vi "DVS_LabVIEWController_april2015 - Copy.vi"() -> ()   [LabVIEW 2013]
doc: "This example demonstrates temperature control and monitoring.\n\nNote:\nBefore start this VI is it necessary:\n\n- preconfigure some specific parameters that are not supported by this driver (e.g. PV-I/O Type, Linearization type, Alarm Input Values... ) by Quick Codes, or by Eurotherm iTools or by instrument front panel controls\n- enter correct VISA Resource Descriptor, Device Address and Baud Rate into front-panel controls"
uses:
  <vilib>/Utility/file.llb/Write To Spreadsheet File (string).vi
  <vilib>/Instr/_visa.llb/VISA Configure Serial Port (Instr).vi
  <instrlib>/Keithley 6430/Public/Data/Read (Single Point).vi
  <instrlib>/Keithley 24XX/Public/Data/Read (Single Point).vi
  <instrlib>/Keithley 24XX/Keithley 24XX.lvlib
  <instrlib>/Keithley 6430/Keithley 6430.lvlib
panel:
  out "(Ohm)":dbl format="%^_7e"
  out "Waveform Chart 9":cluster{"Measurement":dbl}(graph)
  in  "Keithley 6430":bool
  in  "Keithley 2422":bool
  in  "Keithley 2423":bool
  in  "Keithley 2421":bool
  in  "stop":bool
  in  "Keithley 2420":bool
  in  "J-KEM":bool
  out "Start Time":string
  out "Elapsed (min)":dbl caption="Elapsed Time (s)"
  out "Data\nfile\npath":path
  in  "Comments":string
  out "Program Errors":errorcluster
  in  "Delay between data points (s)":dbl format="%#_13g"
  in  "Stop after (min)":dbl
  in  "Auto stop?":bool
  out "Tot. mass (g)":dbl
  out "F_o (MHz)":dbl
  out "Waveform Chart 8":cluster{dbl}(graph)
  out "Ohm":dbl format="%.4e"
  out "MHz":dbl format="%.6f"
  out "Waveform Chart 7":cluster{dbl, "Resistance out":dbl}(graph)
  out "°C":dbl
  out "Waveform Chart 5":cluster{dbl}(graph)
  out "Ohm":sgl
  out "Waveform Chart 4":cluster{"Resistance":sgl}(graph)
  in  "Clear all charts":bool
  out "Waveform Chart 6":cluster{dbl}(graph)
  out "O2 Concentration (PPM)":dbl
  out "Waveform Chart":cluster{dbl}(graph)
  out "Torr":dbl
  out "%":dbl
  out "atm":dbl
  in  "Com Port":i32(ring) items=["Com 1", "Com 2", "Com 3", "Com 4", "Com 5", "Com 6", "COM 7", "COM 8", "COM 9", "COM 10", "COM 11", "COM 12", "com 13", "COM 14"]
  in  "Baud Rate 2":i32(ring)=2 items=["2400", "4800", "9600", "19200", "38400", "57600", "115200"]
  in  "Com Port 2":i32(ring) items=["Com 1", "Com 2", "Com 3", "Com 4", "Com 5", "Com 6", "COM 7", "COM 8", "COM 9", "COM 10", "COM 11", "COM 12", "com 13", "COM 14"]
  # "Configuring Instrument\n \nPlease Wait......\n\nChart will update in 20 sec"
  # "Sample Temperature"
  # "O2 Partial Pressure"
  # "SetNag\nO2 Pump"
  # "Rapidox O2 Sensor"
  # "Keithley 6430 Resistance"
  # "Setup"
  # "Instruments Connected:"
  # "Timing"
  # "SRS QCM"
  # "Keithley 2420 Resistance"
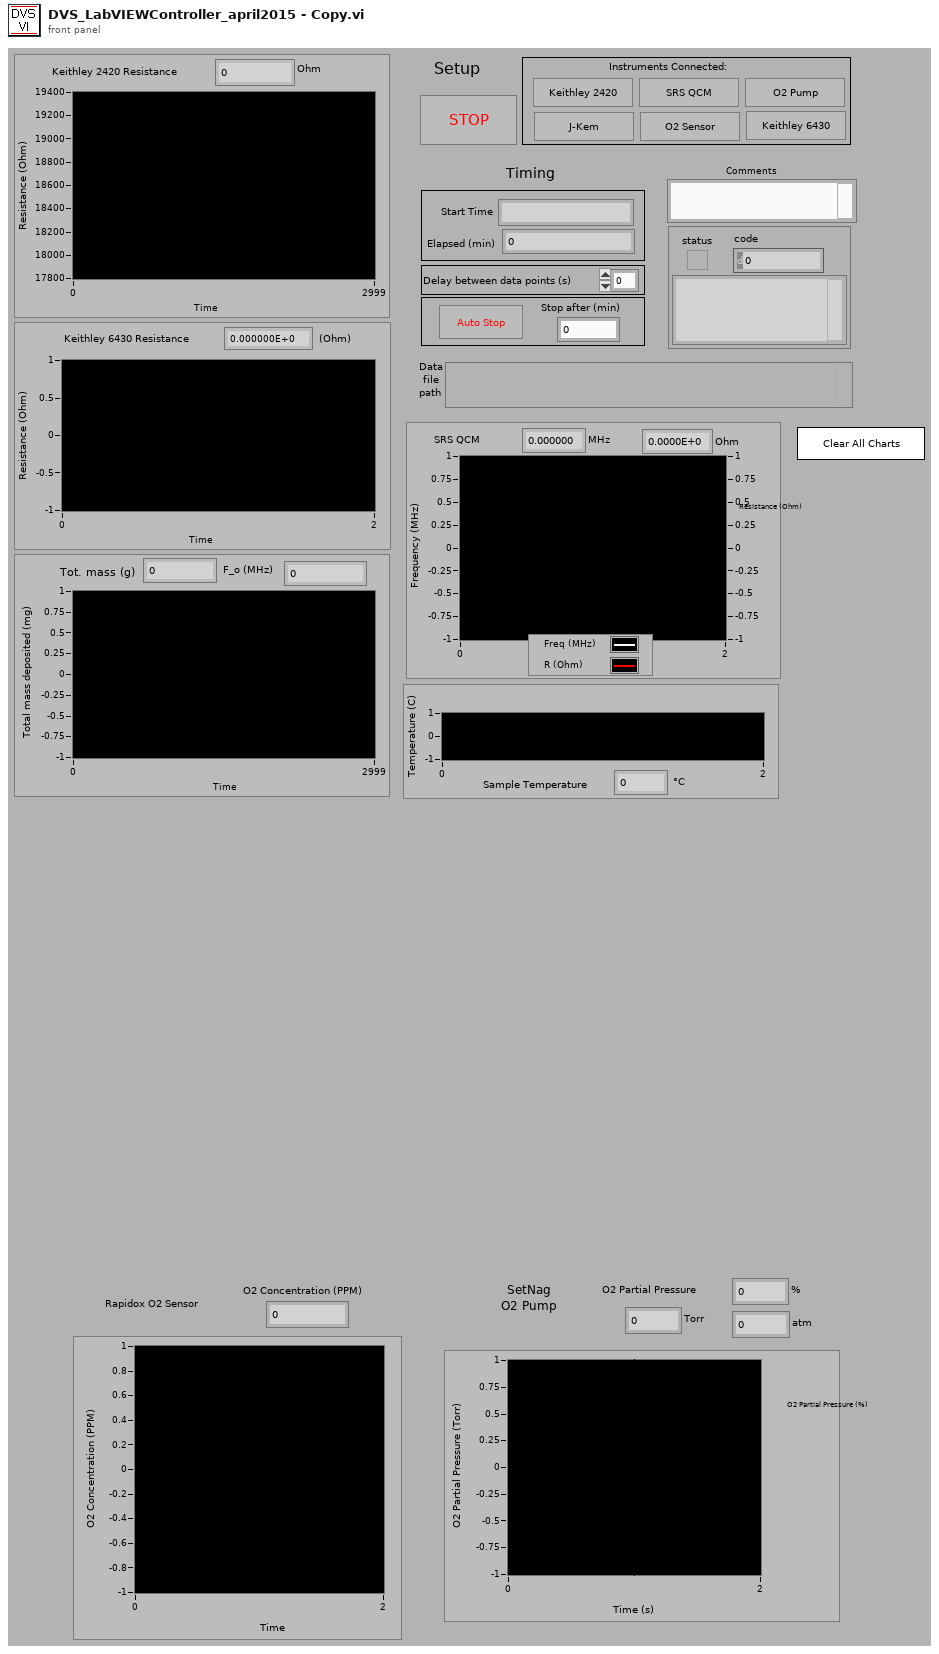
[diagram p1: front panel]
types:
  T1 = enum16{"open", "open or create", "create or replace", "create", "open (read only)"}
  T2 = cluster{"Baud Rate":u32, "Parity":u16, "Data Bits":u16, "Stop Bits":u16, "Flow Control":u16}
  T3 = enum16{"no parity", "odd parity", "even parity", "mark parity", "space parity"}
  T4 = cluster{bool, "VISA resource name":refnum<visa-resource-name>, "error out":errorcluster}
  T5 = cluster{bool, "VISA resource name out":refnum<visa-resource-name>, "error out":errorcluster}
  T6 = cluster{bool, "VISA out":refnum<visa-resource-name>, "error out":errorcluster}
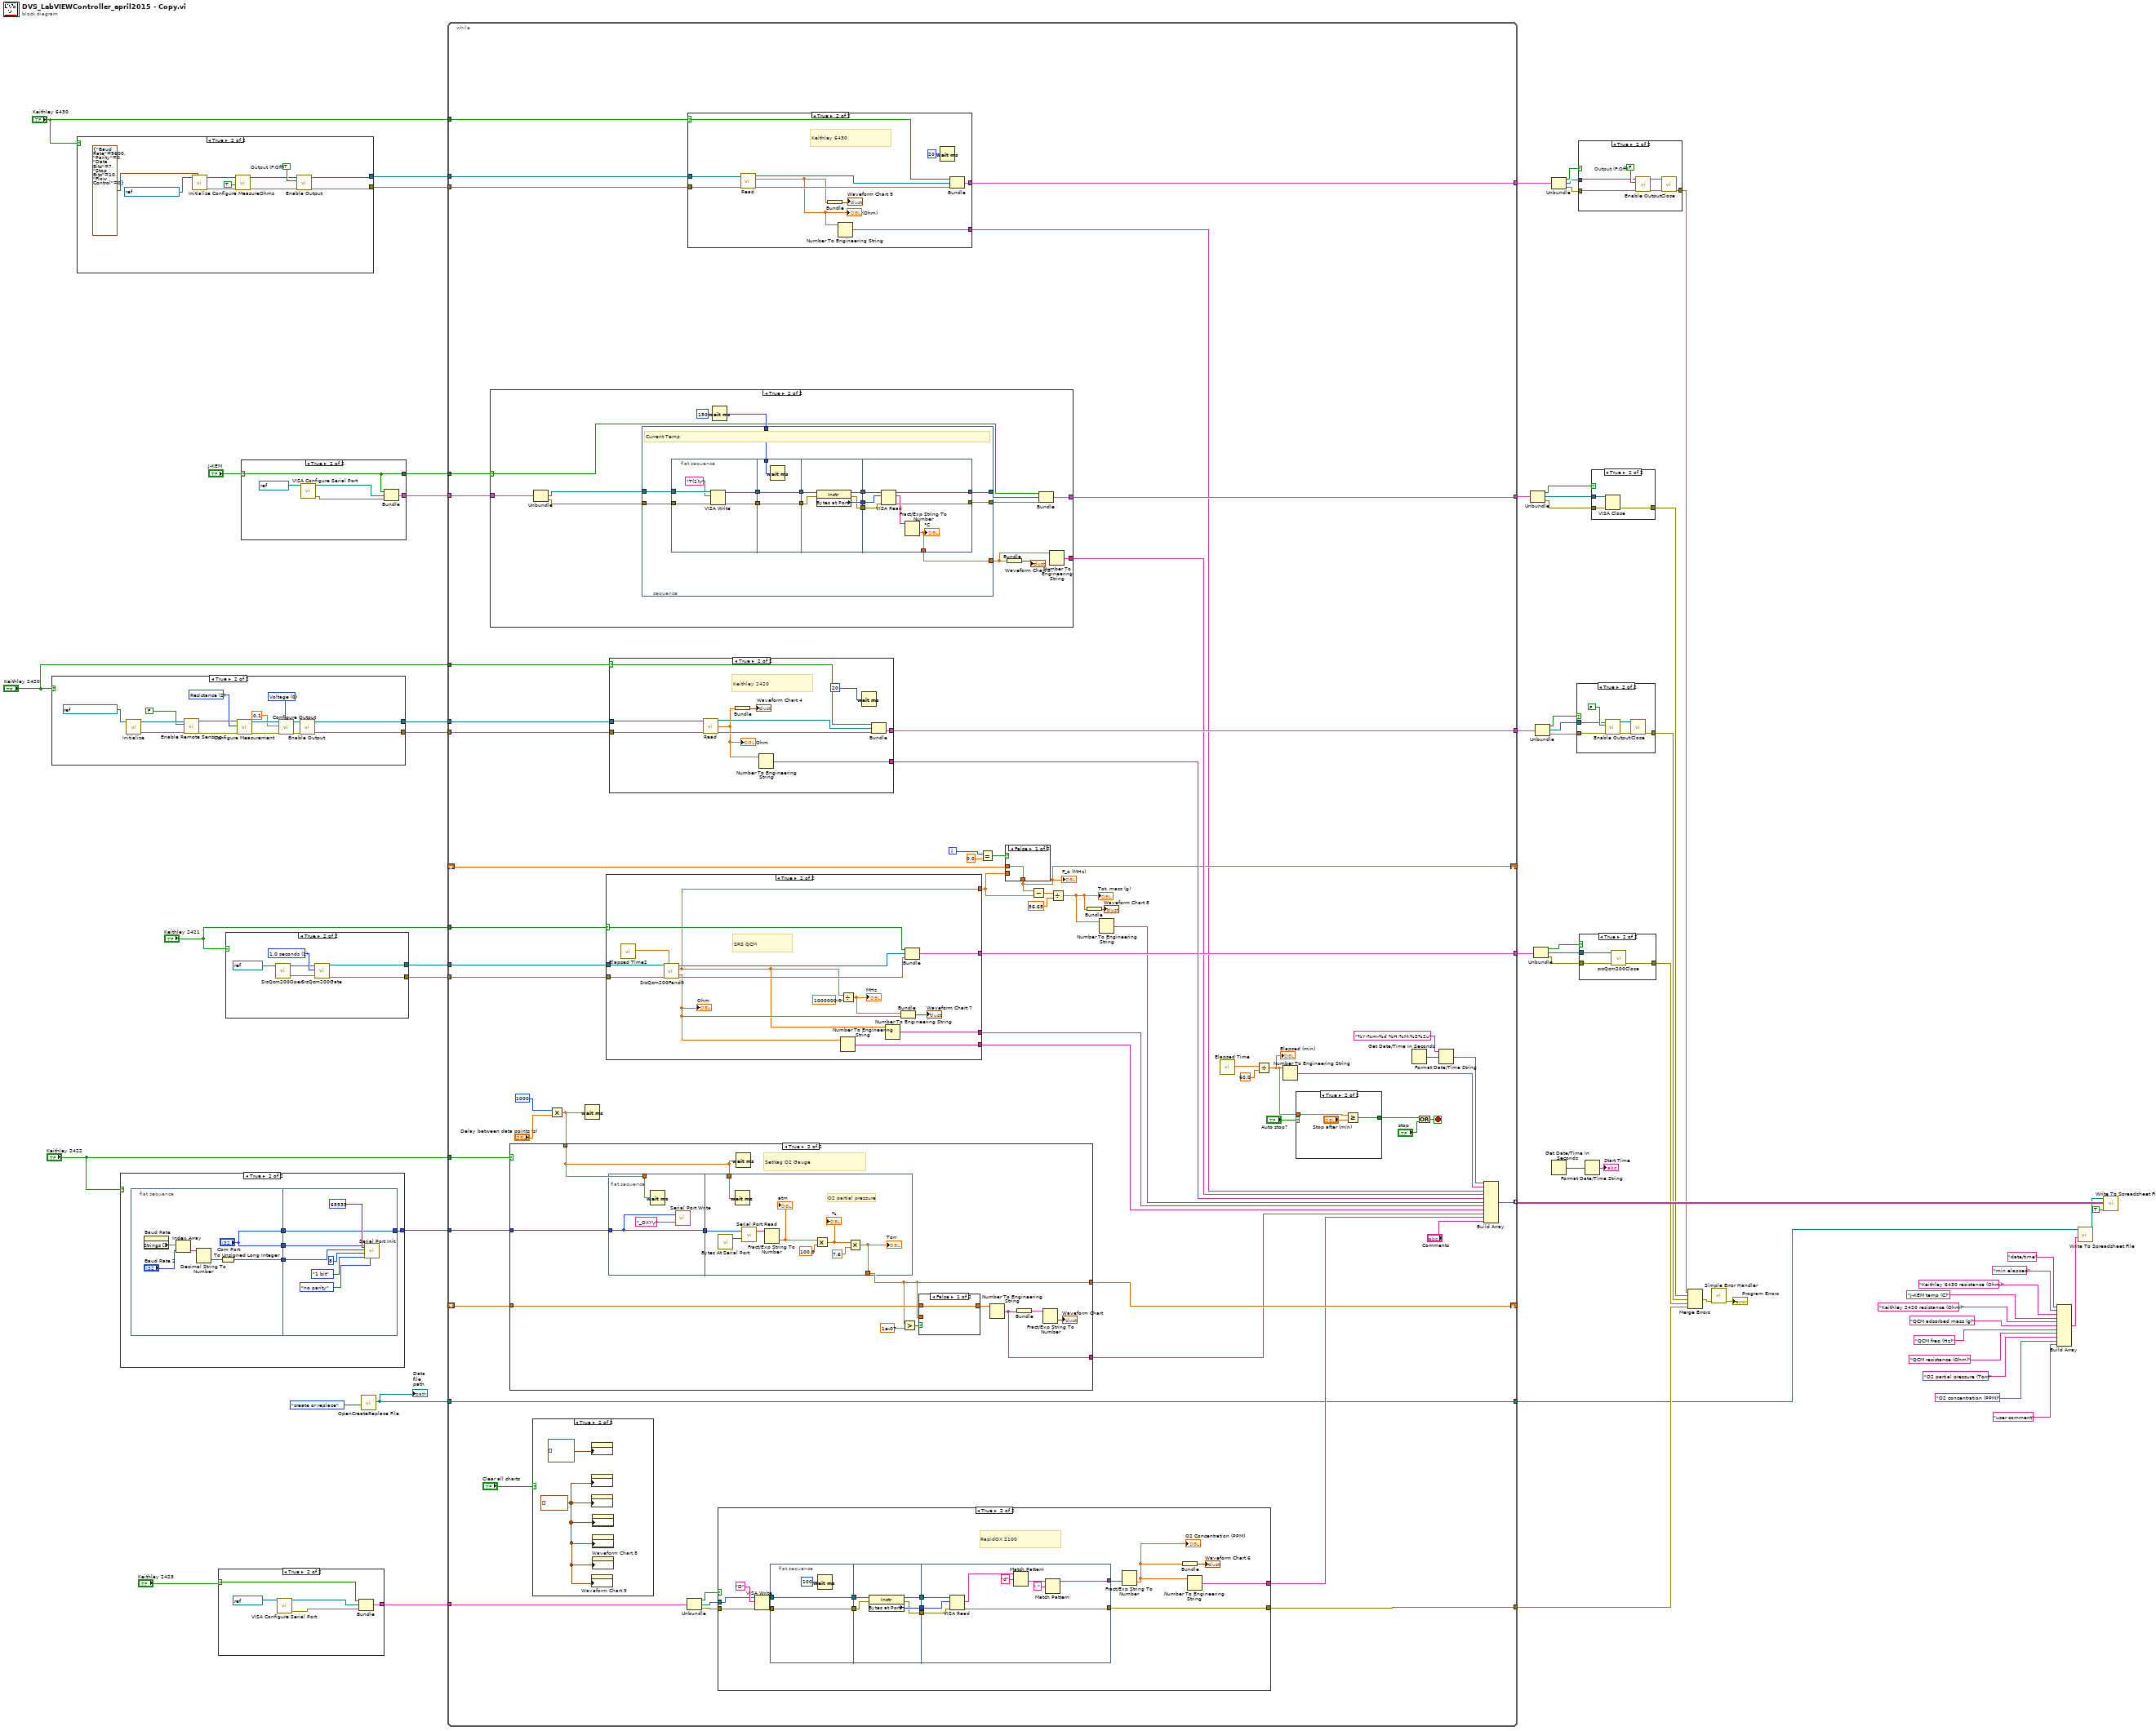
[diagram p0: block diagram]
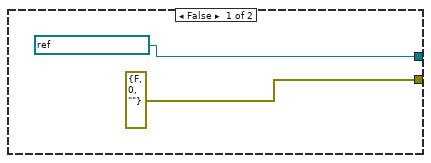
[diagram p3: hidden frame]
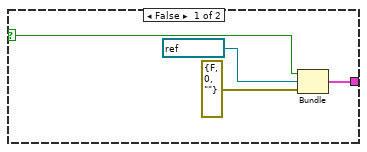
[diagram p4: hidden frame]
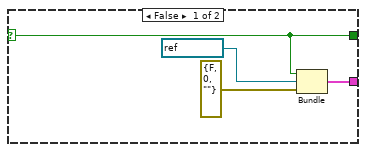
[diagram p6: hidden frame]
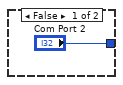
[diagram p7: hidden frame]
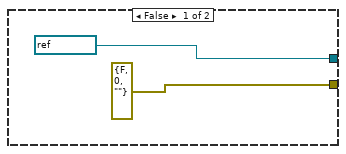
[diagram p9: hidden frame]
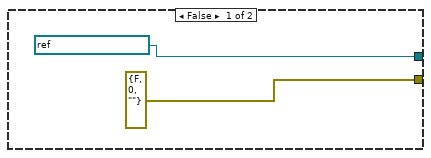
[diagram p11: hidden frame]
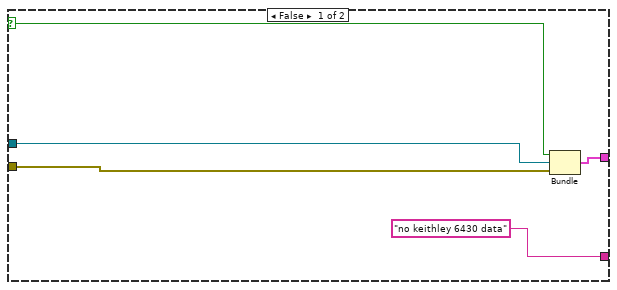
[diagram p12: hidden frame]
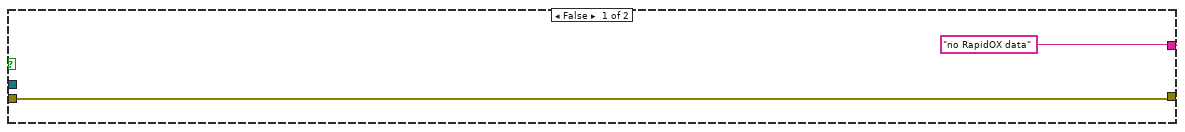
[diagram p15: hidden frame]
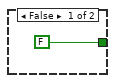
[diagram p16: hidden frame]
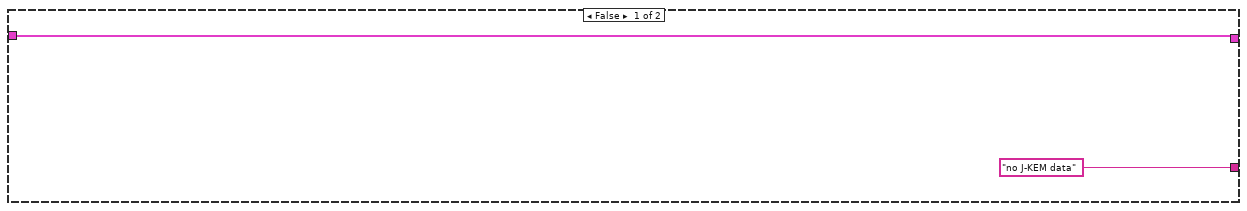
[diagram p17: hidden frame]
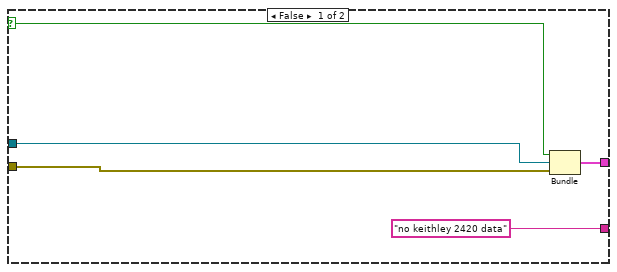
[diagram p18: hidden frame]
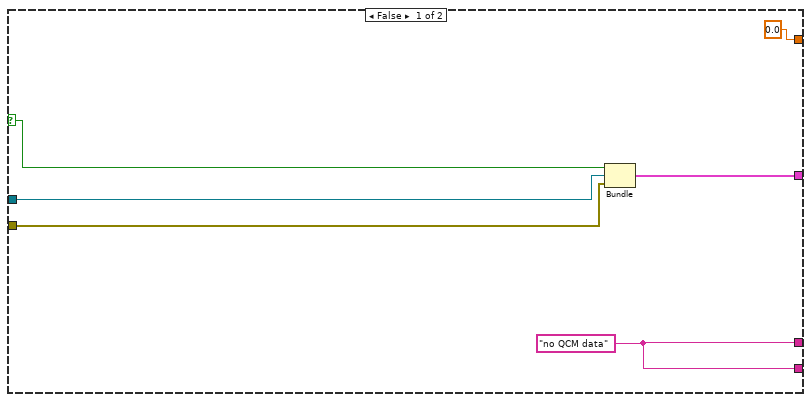
[diagram p19: hidden frame]
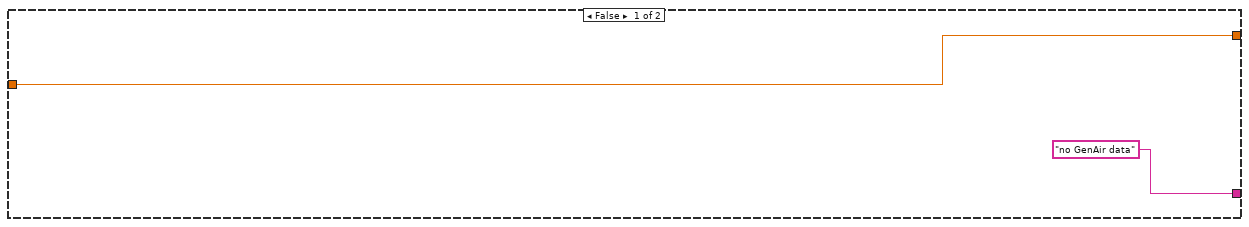
[diagram p20: hidden frame]
diagram:
  n1 = case shown="True" "Keithley 2420" {
    tunnel: [refnum<visa-resource-name> "GPIB1::24::INSTR" ("VISA resource name") w68] -> w54
    tunnel: [errorcluster {"status"=FALSE, "code"=0, "source"=""} ("error out") w63] -> w53
    frame False {
    }
    frame True {
      w70 = u16 0 items=["Voltage", "Current"] ("Source Mode  (0: Voltage)")
      w75 = u16 2 items=["Volts", "Current", "Resistance"] ("Function (0: Volts)")
      n2 = call <instrlib>:"Initialize.vi"("VISA resource name"=refnum<visa-resource-name> "GPIB1::24::INSTR") -> ("error out"=w64:errorcluster, "VISA resource name out"=w67:refnum<visa-resource-name>)  [unwired: 9 in]
      n3 = call <instrlib>:"Enable Remote Sensing.vi"("error in (no error)"=w64, "Enable Remote Sensing (T: Enable)"=FALSE ("4-wire?"), "VISA resource name"=w67) -> ("error out"=w65:errorcluster, "VISA resource name out"=w66:refnum<visa-resource-name>)  [unwired: 7 in]
      n4 = call <instrlib>:"Configure Measurement.vi"("error in (no error)"=w65, "Function (0: Volts)"=w75, "VISA resource name"=w66) -> ("error out"=w74:errorcluster, "VISA resource name out"=w73:refnum<visa-resource-name>)  [unwired: 7 in]
      n5 = call <instrlib>:"Configure Output.vi"("Source Mode  (0: Voltage)"=w70, "error in (no error)"=w74, "Output Level (0)"=0.1 ("Applied Voltage (V)"), "VISA resource name"=w73) -> ("error out"=w72:errorcluster, "VISA resource name out"=w71:refnum<visa-resource-name>)  [unwired: 6 in]
      n6 = call <instrlib>:"Enable Output.vi"("error in (no error)"=w72, "VISA resource name"=w71) -> ("error out"=w63:errorcluster, "VISA resource name out"=w68:refnum<visa-resource-name>)  [unwired: 8 in]
    }
  }
  n7 = case shown="True" "Keithley 6430" {
    tunnel: [refnum<visa-resource-name> "GPIB0::29::INSTR" ("VISA resource name") w80] -> w6
    tunnel: [errorcluster {"status"=FALSE, "code"=0, "source"=""} ("error out") w81] -> w5
    frame False {
    }
    frame True {
      w87 = TRUE  # Output (F:Off)
      n8 = call <instrlib>:"Initialize.vi"("Serial Configuration"=T2 {"Baud Rate"=9600, "Parity"=0, "Data Bits"=7, "Stop Bits"=10, "Flow Control"=0}, "VISA resource name"=refnum<visa-resource-name> "GPIB0::29::INSTR") -> ("error out"=w84:errorcluster, "VISA resource name out"=w83:refnum<visa-resource-name>)  [unwired: 3 in, 5 out]
      n9 = call <instrlib>:"Configure MeasureOhms.vi"("error in (no error)"=w84, "Auto Range (T:Enable)"=TRUE, "VISA resource name"=w83) -> ("error out"=w88:errorcluster, "VISA resource name out"=w85:refnum<visa-resource-name>)  [unwired: 3 in, 4 out]
      n10 = call <instrlib>:"Enable Output.vi"("error in (no error)"=w88, "Enable Output (F:Off)"=w87, "VISA resource name"=w85) -> ("error out"=w81:errorcluster, "VISA resource name out"=w80:refnum<visa-resource-name>)  [unwired: 7 out]
    }
  }
  n11 = case shown="True" "Keithley 2422" {
    tunnel: ["Com Port 2" w90] -> w50
    frame False {
    }
    frame True {
      n12 = flat-sequence {
        tunnel: ["Com Port"] -> w93
        tunnel: [w95] -> w92
        tunnel: ["Com Port"] -> w91
        tunnel: w93 -> [w101]
        tunnel: w92 -> [w100]
        tunnel: w91 -> [w102]
        tunnel: [w102] -> w90
        frame #0 {
          n13 = property on="Baud Rate" class="Ring (strict)"() -> ("Strings []"=w97:string[])  [unwired: 2 in, 2 out]
          n14 = Index Array(array=w97, index="Baud Rate 2") -> (element=w98:string)
          n15 = Decimal String To Number(string=w98) -> (number=w96:i32)  [unwired: 2 in, 1 out]
          n16 = To Unsigned Long Integer(number=w96) -> (unsigned 32bit integer=w95:u32)
        }
        frame #1 {
          n17 = call <vilib>:"Serial Port Init.vi"("parity"=T3."no parity", "buffer size"=u16 65535, "stop bits"=enum16{"1 bit", "1.5 bits", "2 bits"}."1 bit", "data bits"=u16 8, "baud rate"=w100, "port number"=w101) -> ()  [unwired: 1 in, 1 out]
        }
      }
    }
  }
  n18 = case shown="True" "Keithley 2423" {
    selector: "Keithley 2423" -> [w107 w112]
    tunnel: [w108 w113] -> w19
    frame False {
      n19 = Bundle(w107, "VISA resource name"=refnum<visa-resource-name> "COM7", "error out"=errorcluster {"status"=FALSE, "code"=0, "source"=""}) -> (w108:T4)  [unwired: 1 in]
    }
    frame True {
      n20 = call-poly "VISA Configure Serial Port"("VISA resource name"=refnum<visa-resource-name> "COM7") -> ("VISA resource name out"=w114:refnum<visa-resource-name>, "error out"=w111:errorcluster)  [unwired: 13 in]
      n21 = Bundle(w112, "VISA resource name out"=w114, "error out"=w111) -> (w113:T5)  [unwired: 1 in]
    }
  }
  n22 = case shown="True" "Keithley 2421" {
    tunnel: [refnum<visa-resource-name> "COM6" ("VISA in") w119] -> w52
    tunnel: [errorcluster {"status"=FALSE, "code"=0, "source"=""} ("error out") w118] -> w51
    frame False {
    }
    frame True {
      w123 = u16 1 items=["0.1 seconds", "1.0 seconds", "10.0 seconds"] ("Gate in")
      n23 = call <instrlib>:"SrsQcm200Open.vi"("VISA in"=refnum<visa-resource-name> "COM6") -> ("error out"=w120:errorcluster, "VISA out"=w121:refnum<visa-resource-name>)  [unwired: 4 in]
      n24 = call <instrlib>:"SrsQcm200Gate.vi"("VISA in"=w121, "Gate in"=w123, "error in (no error)"=w120) -> ("VISA out"=w119:refnum<visa-resource-name>, "error out"=w118:errorcluster)  [unwired: 14 in, 1 out]
    }
  }
  n25 = case shown="True" "J-KEM" {
    selector: "J-KEM" -> [w124 w129]
    tunnel: [w125 w130] -> w39
    tunnel: [w124 w129] -> w32
    frame False {
      n26 = Bundle(w124, "VISA resource name"=refnum<visa-resource-name> "COM3", "error out"=errorcluster {"status"=FALSE, "code"=0, "source"=""}) -> (w125:T4)  [unwired: 1 in]
    }
    frame True {
      n27 = call-poly "VISA Configure Serial Port"("VISA resource name"=refnum<visa-resource-name> "COM3") -> ("VISA resource name out"=w131:refnum<visa-resource-name>, "error out"=w128:errorcluster)  [unwired: 13 in]
      n28 = Bundle(w129, "VISA resource name out"=w131, "error out"=w128) -> (w130:T5)  [unwired: 1 in]
    }
  }
  n29 = call <instrlib>:"OpenCreateReplace File.vi"("function (open:0)"=T1."create or replace") -> ("new file path"=w15:path)  [unwired: 7 in, 3 out]
  "Data\nfile\npath" <- w15
  n30 = while {
    shift-right: [w190] -> _
    shift-left: _ -> [w189]
    tunnel: [w187] -> w56 mode=indexing
    tunnel: "Keithley 2420" -> [w153]
    tunnel: w54 -> [w185]
    tunnel: w53 -> [w184]
    tunnel: w52 -> [w183]
    tunnel: w51 -> [w182]
    tunnel: "Keithley 2421" -> [w180]
    tunnel: "Keithley 2422" -> [w173]
    tunnel: w50 -> [w179]
    tunnel: [w175] -> w47
    tunnel: [w174] -> w43
    tunnel: w39 -> [w172]
    tunnel: [w171] -> w37
    tunnel: w32 -> [w169]
    tunnel: w19 -> [w162]
    tunnel: [w157] -> w17
    tunnel: [w152] -> w16
    tunnel: w15 -> [w152]
    shift-right: [w141] -> _
    shift-left: _ -> [w140]
    tunnel: w6 -> [w139]
    tunnel: w5 -> [w138]
    tunnel: [w137] -> w3
    tunnel: "Keithley 6430" -> [w136]
    i -> [w148]
    stop <- w167 stop-if-true
    n31 = case shown="True" w169 {
      selector: w169 -> [_ w253]
      tunnel: w172 -> [w251 w258]
      tunnel: [w251 w256] -> w171
      tunnel: ["no J-KEM data" w254] -> w170
      frame False {
      }
      frame True {
        w262 = u32 150 ("milliseconds to wait")
        n32 = Unbundle(w258) -> ("VISA resource name out"=w257:refnum<visa-resource-name>, "error out"=w252:errorcluster)  [unwired: 1 out]
        n33 = stacked-sequence {
          tunnel: w257 -> [w268]
          tunnel: w252 -> [w267]
          tunnel: w262 -> [w266]
          tunnel: [w264] -> w259
          tunnel: [w263] -> w260
          tunnel: [w265] -> w255
          frame #0 {
            # "Current Temp"
            n34 = flat-sequence {
              tunnel: w268 -> [w280]
              tunnel: w267 -> [w279]
              tunnel: [w277] -> w275
              tunnel: [w276] -> w274
              tunnel: w266 -> [w283]
              tunnel: [w282] -> w273
              tunnel: w275 -> [w282]
              tunnel: w274 -> [w281]
              tunnel: [w281] -> w272
              tunnel: w273 -> [w288]
              tunnel: w272 -> [w287]
              tunnel: [w286] -> w271
              tunnel: [w285] -> w270
              tunnel: [w284] -> w269
              tunnel: w271 -> [w295]
              tunnel: w270 -> [w294]
              tunnel: w269 -> [w293]
              tunnel: [w290] -> w263
              tunnel: [w291] -> w264
              tunnel: [w289] -> w265
              frame #0 {
                n35 = VISA Write(VISA resource name=w280, write buffer="T(1)\r", error in (no error)=w279) -> (VISA resource name out=w277:refnum<visa-resource-name>, error out=w276:errorcluster)  [unwired: 1 out]
              }
              frame #1 {
                n36 = Wait (ms)(milliseconds to wait=w283) -> ()  [unwired: 1 out]
              }
              frame #2 {
                n37 = property class="Instr"(reference=w288, error in=w287) -> (reference out=w286:refnum<visa-resource-name>, error out=w284:errorcluster, "Bytes at Port"=w285:u32)
              }
              frame #3 {
                n38 = VISA Read(VISA resource name=w295, byte count=w294, error in (no error)=w293) -> (VISA resource name out=w291:refnum<visa-resource-name>, read buffer=w292:string, error out=w290:errorcluster)  [unwired: 1 out]
                n39 = Fract/Exp String To Number(string=w292) -> (number=w289:dbl)  [unwired: 3 in, 1 out]
                "°C" <- w289
              }
            }
          }
        }
        n40 = Wait (ms)(milliseconds to wait=w262) -> ()  [unwired: 1 out]
        n41 = Bundle(w255) -> (→"Waveform Chart 5":cluster{dbl})  [unwired: 1 in]
        n42 = Bundle(w253, "VISA resource name out"=w259, "error out"=w260) -> (w256:T5)  [unwired: 1 in]
        n43 = Number To Engineering String(4:w255) -> (0:w254:string)  [unwired: 3 in]
      }
    }
    n44 = case shown="True" "Clear all charts" {
      frame False {
      }
      frame True {
        w210 = cluster{dbl}[] [] ("History Data")
        n45 = property on="Waveform Chart 7" class="WFChart (strict)"("History Data"=cluster{dbl, "Resistance out":dbl}[] []) -> ()  [unwired: 2 in, 2 out]
        n46 = property on="Waveform Chart 4" class="WFChart (strict)"("History Data"=w210) -> ()  [unwired: 2 in, 2 out]
        n47 = property on="Waveform Chart 5" class="WFChart (strict)"("History Data"=w210) -> ()  [unwired: 2 in, 2 out]
        n48 = property on="Waveform Chart 9" class="WFChart (strict)"("History Data"=w210) -> ()  [unwired: 2 in, 2 out]
        n49 = property on="Waveform Chart" class="WFChart (strict)"("History Data"=w210) -> ()  [unwired: 2 in, 2 out]
        n50 = property on="Waveform Chart 6" class="WFChart (strict)"("History Data"=w210) -> ()  [unwired: 2 in, 2 out]
        n51 = property on="Waveform Chart 8" class="WFChart (strict)"("History Data"=w210) -> ()  [unwired: 2 in, 2 out]
      }
    }
    n52 = Multiply(x=u32 1000, y="Delay between data points (s)") -> (x*y=w156:dbl)
    n53 = case shown="True" w173 {
      tunnel: [w332 w336] -> w190
      tunnel: w189 -> [w332 w337]
      tunnel: w156 -> [_ w333]
      tunnel: w179 -> [_ w335]
      tunnel: ["no GenAir data" w334] -> w178
      frame False {
      }
      frame True {
        # "SetNag O2 Gauge"
        n54 = flat-sequence {
          tunnel: [w346] -> w343
          tunnel: w333 -> [w348]
          tunnel: w335 -> [w346]
          tunnel: w343 -> [w349]
          tunnel: w333 -> [w356]
          tunnel: [w352] -> w336
          frame #0 {
            n55 = Wait (ms)(milliseconds to wait=w348) -> ()  [unwired: 1 out]
            n56 = call <vilib>:"Serial Port Write.vi"("string to write"="_OXY\r" ("O2 partial press"), "port number"=w346) -> ()  [unwired: 1 out]
          }
          frame #1 {
            # "O2 partial pressure"
            n57 = call <vilib>:"Bytes At Serial Port.vi"() -> ("byte count"=w357:u32)  [unwired: 1 in, 1 out]
            n58 = Wait (ms)(milliseconds to wait=w356) -> ()  [unwired: 1 out]
            n59 = call <vilib>:"Serial Port Read.vi"("requested byte count"=w357, "port number"=w349) -> ("string read"=w355:string)  [unwired: 1 out]
            n60 = Fract/Exp String To Number(string=w355) -> (number=w353:dbl)  [unwired: 3 in, 1 out]
            "atm" <- w353
            n61 = Multiply(x=w353, y=100.0) -> (x*y=w350:dbl)
            "%" <- w350
            n62 = Multiply(x=w350, y=7.6) -> (x*y=w352:dbl)
            "Torr" <- w352
          }
        }
        n63 = Wait (ms)(milliseconds to wait=w333) -> ()  [unwired: 1 out]
        n64 = Greater?(x=w336, y=1e-07) -> (0:w339:bool)
        n65 = case shown="False" w339 {
          tunnel: [w344 w345] -> w338
          tunnel: w336 -> [_ w345]
          tunnel: w337 -> [w344 _]
          frame False {
          }
          frame True {
          }
        }
        n66 = Number To Engineering String(4:w338) -> (0:w334:string)  [unwired: 3 in]
        n67 = Bundle(w334) -> (w341:cluster{string})  [unwired: 1 in]
        n68 = Fract/Exp String To Number(string=w341) -> (number=→"Waveform Chart":cluster{dbl})  [unwired: 3 in, 1 out]
      }
    }
    n69 = Wait (ms)(milliseconds to wait=w156) -> ()  [unwired: 1 out]
    n70 = case shown="True" w180 {
      selector: w180 -> [w315 w328]
      tunnel: w183 -> [w314 w322]
      tunnel: w182 -> [w313 w324]
      tunnel: [w316 w330] -> w181
      tunnel: [w316 w329] -> w177
      tunnel: [w312 w327] -> w174
      tunnel: [0.0 w317] -> w144
      frame False {
        w316 = "no QCM data"
        n71 = Bundle(w315, "VISA out"=w314, "error out"=w313) -> (w312:T6)  [unwired: 1 in]
      }
      frame True {
        # "SRS QCM"
        n72 = call "Elapsed Time2"() -> ("Elapsed Time (s)"=w323:dbl)  [unwired: 12 in, 7 out]
        n73 = call <instrlib>:"SrsQcm200FandR.vi"("VISA in"=w322, "Reference time in"=w323, "error in (no error)"=w324) -> ("VISA out"=w320:refnum<visa-resource-name>, "Frequency out"=w317:dbl, "Resistance out"=w319:dbl, "error out"=w321:errorcluster)  [unwired: 6 in, 3 out]
        "Ohm" <- w319
        n74 = Number To Engineering String(4:w319) -> (0:w329:string)  [unwired: 3 in]
        n75 = Divide(x=w317, y=1000000.0) -> (x/y=w318:dbl)
        "MHz" <- w318
        n76 = Number To Engineering String(4:w317) -> (0:w330:string)  [unwired: 3 in]
        n77 = Bundle(w318, "Resistance out"=w319) -> (→"Waveform Chart 7":cluster{dbl, "Resistance out":dbl})  [unwired: 1 in]
        n78 = Bundle(w328, "VISA out"=w320, "error out"=w321) -> (w327:T6)  [unwired: 1 in]
      }
    }
    n79 = case shown="True" w153 {
      selector: w153 -> [w299 w307]
      tunnel: w185 -> [w298 w302]
      tunnel: w184 -> [w297 w301]
      tunnel: [w296 w305] -> w175
      tunnel: ["no keithley 2420 data" w304] -> w176
      frame False {
        n80 = Bundle(w299, "VISA resource name out"=w298, "error out"=w297) -> (w296:T5)  [unwired: 1 in]
      }
      frame True {
        # "Keithley 2420"
        n81 = call-poly <instrlib>:"Read.vi"("VISA resource name"=w302, "error in (no error)"=w301) -> ("VISA resource name out"=w308:refnum<visa-resource-name>, "Resistance"=w303:sgl, "error out"=w306:errorcluster)  [unwired: 7 in, 4 out]
        "Ohm" <- w303
        n82 = Bundle("Resistance"=w303) -> (→"Waveform Chart 4":cluster{"Resistance":sgl})  [unwired: 1 in]
        n83 = Number To Engineering String(4:w303) -> (0:w304:string)  [unwired: 3 in]
        n84 = Wait (ms)(milliseconds to wait=u32 20) -> ()  [unwired: 1 out]
        n85 = Bundle(w307, "VISA resource name out"=w308, "error out"=w306) -> (w305:T5)  [unwired: 1 in]
      }
    }
    n86 = Unbundle(w162) -> (w161:bool, "VISA resource name out"=w160:refnum<visa-resource-name>, "error out"=w159:errorcluster)
    n87 = case shown="True" w136 {
      selector: w136 -> [w196 w206]
      tunnel: w139 -> [w195 w203]
      tunnel: w138 -> [w194 w202]
      tunnel: ["no keithley 6430 data" w205] -> w135
      tunnel: [w193 w204] -> w137
      frame False {
        n88 = Bundle(w196, "VISA resource name out"=w195, "error out"=w194) -> (w193:T5)  [unwired: 1 in]
      }
      frame True {
        # "Keithley 6430"
        n89 = call-poly <instrlib>:"Read.vi"("error in (no error)"=w202, "VISA resource name"=w203) -> ("error out"=w201:errorcluster, "Measurement"=w199:dbl, "VISA resource name out"=w200:refnum<visa-resource-name>)  [unwired: 1 in, 6 out]
        "(Ohm)" <- w199
        n90 = Bundle("Measurement"=w199) -> (→"Waveform Chart 9":cluster{"Measurement":dbl})  [unwired: 1 in]
        n91 = Number To Engineering String(4:w199) -> (0:w205:string)  [unwired: 3 in]
        n92 = Wait (ms)(milliseconds to wait=u32 20) -> ()  [unwired: 1 out]
        n93 = Bundle(w206, "VISA resource name out"=w200, "error out"=w201) -> (w204:T5)  [unwired: 1 in]
      }
    }
    n94 = case shown="True" w161 {
      tunnel: w160 -> [_ w219]
      tunnel: w159 -> [w212 w218]
      tunnel: ["no RapidOX data" w217] -> w158
      tunnel: [w212 w214] -> w157
      frame False {
      }
      frame True {
        # "RapidOX 2100"
        n95 = VISA Write(VISA resource name=w219, write buffer="D", error in (no error)=w218) -> (VISA resource name out=w222:refnum<visa-resource-name>, error out=w221:errorcluster)  [unwired: 1 out]
        n96 = flat-sequence {
          tunnel: [w231] -> w228
          tunnel: [w229] -> w227
          tunnel: w222 -> [w231]
          tunnel: w221 -> [w229]
          tunnel: w228 -> [w236]
          tunnel: w227 -> [w235]
          tunnel: [w234] -> w226
          tunnel: [w233] -> w225
          tunnel: [w232] -> w224
          tunnel: w226 -> [w245]
          tunnel: w225 -> [w244]
          tunnel: w224 -> [w243]
          tunnel: [w242] -> w214
          tunnel: [w237] -> w216
          frame #0 {
            n97 = Wait (ms)(milliseconds to wait=u32 100) -> ()  [unwired: 1 out]
          }
          frame #1 {
            n98 = property class="Instr"(reference=w236, error in=w235) -> (reference out=w234:refnum<visa-resource-name>, error out=w232:errorcluster, "Bytes at Port"=w233:u32)
          }
          frame #2 {
            n99 = VISA Read(VISA resource name=w245, byte count=w244, error in (no error)=w243) -> (read buffer=w240:string, error out=w242:errorcluster)  [unwired: 2 out]
            n100 = Match Pattern(string=w240, regular expression="d") -> (after substring=w238:string)  [unwired: 1 in, 3 out]
            n101 = Match Pattern(string=w238, regular expression=",") -> (before substring=w237:string)  [unwired: 1 in, 3 out]
          }
        }
        n102 = Fract/Exp String To Number(string=w216) -> (number=w215:dbl)  [unwired: 3 in, 1 out]
        "O2 Concentration (PPM)" <- w215
        n103 = Bundle(w215) -> (→"Waveform Chart 6":cluster{dbl})  [unwired: 1 in]
        n104 = Number To Engineering String(4:w215) -> (0:w217:string)  [unwired: 3 in]
      }
    }
    n105 = Equal?(x=w148, y=0.0) -> (x = y?=w147:bool)
    n106 = case shown="False" w147 {
      tunnel: w144 -> [_ w209]
      tunnel: [w208 w209] -> w141
      tunnel: w140 -> [w208 _]
      frame False {
      }
      frame True {
      }
    }
    "F_o (MHz)" <- w141
    n107 = Subtract(x=w141, y=w144) -> (x-y=w145:dbl)
    n108 = Divide(x=w145, y=56.65) -> (x/y=w134:dbl)
    "Tot. mass (g)" <- w134
    n109 = Bundle(w134) -> (→"Waveform Chart 8":cluster{dbl})  [unwired: 1 in]
    n110 = Number To Engineering String(4:w134) -> (0:w142:string)  [unwired: 3 in]
    n111 = call "Elapsed Time"() -> ("Elapsed Time (s)"=w166:dbl)  [unwired: 12 in, 7 out]
    n112 = Divide(x=w166, y=60.0) -> (x/y=w150:dbl)
    "Elapsed (min)" <- w150
    n113 = Number To Engineering String(4:w150) -> (0:w191:string)  [unwired: 3 in]
    n114 = case shown="True" "Auto stop?" {
      tunnel: [FALSE w249] -> w163
      tunnel: w150 -> [_ w247]
      frame False {
      }
      frame True {
        n115 = Greater Or Equal?(x=w247, y="Stop after (min)") -> (x >= y?=w249:bool)
      }
    }
    n116 = Get Date/Time In Seconds() -> (seconds since 1Jan1904=w192:timestamp)
    n117 = Or(x=w163, y="stop") -> (x .or. y?=w167:bool)
    n118 = Format Date/Time String(time format string (%c)="%Y-%m-%d %H:%M:%S%2u", seconds (now)=w192) -> (date/time string=w186:string)  [unwired: 1 in]
    n119 = Build Array(w186, w191, w135, w170, w176, w142, w181, w177, w178, w158, "Comments") -> (w187:string[])
  }
  n120 = Unbundle(w37) -> (w36:bool, "VISA resource name out"=w35:refnum<visa-resource-name>, "error out"=w34:errorcluster)
  n121 = Unbundle(w43) -> (w42:bool, "VISA out"=w41:refnum<visa-resource-name>, "error out"=w40:errorcluster)
  n122 = Unbundle(w47) -> (w46:bool, "VISA resource name out"=w45:refnum<visa-resource-name>, "error out"=w44:errorcluster)
  n123 = Unbundle(w3) -> (w9:bool, "VISA resource name out"=w8:refnum<visa-resource-name>, "error out"=w7:errorcluster)
  n124 = Get Date/Time In Seconds() -> (seconds since 1Jan1904=w58:timestamp)
  n125 = case shown="True" w46 {
    tunnel: w45 -> [_ w361]
    tunnel: w44 -> [w358 w360]
    tunnel: [w358 w359] -> w48
    frame False {
    }
    frame True {
      n126 = call <instrlib>:"Enable Output.vi"("error in (no error)"=w360, "Enable Output (T: Enable)"=FALSE, "VISA resource name"=w361) -> ("error out"=w362:errorcluster, "VISA resource name out"=w364:refnum<visa-resource-name>)  [unwired: 7 in]
      n127 = call <instrlib>:"Close.vi"("error in (no error)"=w362, "VISA resource name"=w364) -> ("error out"=w359:errorcluster)  [unwired: 9 in]
    }
  }
  n128 = case shown="True" w9 {
    tunnel: w8 -> [_ w367]
    tunnel: w7 -> [w365 w366]
    tunnel: [w365 w368] -> w2
    frame False {
    }
    frame True {
      w371 = FALSE  # Output (F:Off)
      n129 = call <instrlib>:"Enable Output.vi"("error in (no error)"=w366, "Enable Output (F:Off)"=w371, "VISA resource name"=w367) -> ("error out"=w369:errorcluster, "VISA resource name out"=w370:refnum<visa-resource-name>)  [unwired: 7 out]
      n130 = call <instrlib>:"Close.vi"("error in (no error)"=w369, "VISA resource name"=w370) -> ("error out"=w368:errorcluster)  [unwired: 9 out]
    }
  }
  n131 = case shown="True" w42 {
    tunnel: w40 -> [w372 w375]
    tunnel: [w372 w374] -> w49
    tunnel: w41 -> [_ w373]
    frame False {
    }
    frame True {
      n132 = call <instrlib>:"srsQcm200Close.vi"("error in"=w375, "Visa in"=w373) -> ("error out"=w374:errorcluster)  [unwired: 3 in]
    }
  }
  n133 = Format Date/Time String(seconds (now)=w58) -> (date/time string=→"Start Time":string)  [unwired: 2 in]
  n134 = case shown="True" w36 {
    tunnel: w35 -> [_ w379]
    tunnel: w34 -> [w376 w378]
    tunnel: [w376 w377] -> w33
    frame False {
    }
    frame True {
      n135 = VISA Close(VISA resource name=w379, error in (no error)=w378) -> (error out=w377:errorcluster)
    }
  }
  n136 = Merge Errors(w2, w33, w48, w49, w17) -> (w57:errorcluster)
  n137 = call <vilib>:"Simple Error Handler.vi"("error in (no error)"=w57) -> ("error out"=→"Program Errors":errorcluster)  [unwired: 4 in, 4 out]
  n138 = Build Array("date/time", "min elapsed", "Keithley 6430 resistance (Ohm)", "J-KEM temp (C)", "Keithley 2420 resistance (Ohm)" ("element"), "QCM adsorbed mass (g)", "QCM freq (Hz)", "QCM resistance (Ohm)", "O2 partial pressure (Torr)" ("element"), "O2 concentration (PPM)" ("element"), "user comment" ("element")) -> (w24:string[])
  n139 = call-poly <vilib>:"Write To Spreadsheet File.vi"("1D data"=w24, "file path (dialog if empty)"=w16) -> ("new file path (Not A Path if cancelled)"=w25:path)  [unwired: 6 in]
  n140 = call-poly <vilib>:"Write To Spreadsheet File.vi"("append to file? (new file:F)"=TRUE, "2D data"=w56, "file path (dialog if empty)"=w25) -> ()  [unwired: 5 in, 1 out]
